vi "SingleAxisControl.vi"() -> ()   [LabVIEW 2021]
uses:
  Parameters/GetAxisParameterDouble.vi
  Parameters/GetAxisParameterString.vi
  Motion/EnableSingle.vi
  Motion/FaultAckSingle.vi
  Motion/DisableSingle.vi
  Motion/MoveIncSingle.vi
  Motion/FreerunSingle.vi
  Motion/AbortSingle.vi
  Motion/HomeSingle.vi
panel:
  in  "Disconnect?":bool
  in  "taskId":i32(ring)=1 items=["TLibrary", "T01", "T02", "T03", "T04", "T05", "T06", "T07", "T08", "T09", "T10", "T11", "T12", "T13", "T14", "T15", "T16", "T17", "T18", "T19", "T20", "T21", "T22", "T23", "T24", "T25", "T26", "T27", "T28", "T29", "T30", "T31"]
  in  "Abort":bool
  out "do stop":bool
  out "Vel Units":string
  out "Pos Units":string
  in  "stop":bool
  out "Vel Fbk":dbl
  out "Pos Fbk":dbl
  out "Status":string
  in  "Jog Right":bool
  in  "Jog Left":bool
  in  "Distance":dbl=1000.0 min=0.0 max=10.0
  in  "Speed":dbl=5000.0 min=0.0 max=100.0
  in  "Jog":bool
  in  "FaultAck":bool
  in  "Home":bool
  in  "Disable":bool
  in  "Enable":bool
  out "Axis":string
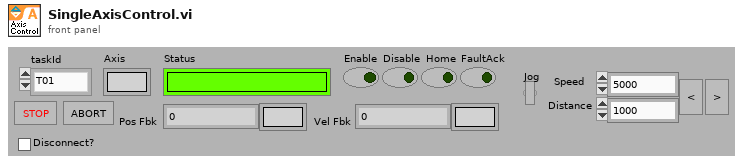
[diagram p1: front panel]
types:
  T1 = cluster{"new reference":refnum<k24>, "Event Callback":refnum<k27>, "ControllerDiagPacket":refnum<user-event>, "Event Registration Refnum":refnum<event-registration>}
  T2 = typedef "AxisDiagPacket.ctl" = cluster{"Axis Name":string, "Analog Input 0":dbl, "Analog Input 1":dbl, "Axis Fault (num)":i32, "Axis Fault (str)":string, "Axis Fault (bits)":cluster{"AmplifierFault":bool, "AmplifierTemperatureFault":bool, "CcwEndOfTravelLimitFault":bool, "CcwSoftwareLimitFault":bool, "CommunicationLostFault":bool, "CwEndOfTravelLimitFault":bool, "CwSoftwareLimitFault":bool, "EmergencyStopFault":bool, "EncoderFault":bool, "ExternalFault":bool, "FeedbackScalingFault":bool, "GantryMisalignFault ":bool, "HallSensorFault":bool, "InPositionTimeoutFault":bool, "MarkerSearchFault":bool, "MaxVelocityCommandFault":bool, "MissedInterruptFault":bool, "MotorTemperatureFault":bool, "None":bool, "OverCurrentFault":bool, "PositionErrorFault":bool, "PositionFeedbackFault":bool, "PowerSupplyFault":bool, "ProbeInputFault":bool, "SafeZoneFault":bool, "VelocityErrorFault":bool, "VelocityFeedbackFault":bool, "VoltageClampFault":bool, "InternalFault":bool}, "Axis Status (num)":i32, "Axis Status (str)":string, "Axis Status (bits)":cluster{"BacklashActive":bool, "CalibrationEnabled1D":bool, "CalibrationEnabled2D":bool, "CommandValid":bool, "DriveAbortPending":bool, "DrivePending":bool, "Enabling":bool, "GainMappingEnabled":bool, "GantryAligned":bool, "GantryRealigning":bool, "Homed":bool, "Homing":bool, "IFOVEnabled":bool, "JogGenerating":bool, "Jogging":bool, "JoystickControl":bool, "MasterSlaveControl":bool, "MotionBlocked":bool, "MotionClamped":bool, "MoveDone":bool, "None":bool, "NotVirtual":bool, "Profiling":bool, "Stability0":bool, "Stability1":bool, "TrajectoryFiltering":bool, "WaitDone":bool}, "Current Command":sgl, "Current Error":sgl, "Current Feedback":sgl, "Digital Inputs":i32, "Digital Outputs":i32, "Drive Status":i32, "Drive Status (str)":string, "Drive Status (bits)":cluster{"AccelerationPhase":bool, "AutofocusActive":bool, "BrakeOutput":bool, "CcwEndOfTravelLimitInput":bool, "CosineEncoderError":bool, "CurrentClamp":bool, "CwEndOfTravelLimitInput":bool, "DecelerationPhase":bool, "DualLoopActive":bool, "EmergencyStopInput":bool, "Enabled":bool, "EncoderClipping":bool, "GalvoCalibrationEnabled":bool, "GalvoPowerCorrection":bool, "HallAInput":bool, "HallBInput":bool, "HallCInput":bool, "HighResolutionMode":bool, "HomeLimitInput":bool, "InPosition":bool, "InPosition2":bool, "MarkerInput":bool, "MarkerLatch":bool, "MoveActive":bool, "NoMotorSupply":bool, "None":bool, "PowerLimiting":bool, "ProgrammingFlash":bool, "ProgrammingMXH":bool, "PSOHaltLatch":bool, "ServoControl":bool, "SineEncoderError":bool}, "Position Feedback Auxiliary":dbl, "Position Command":dbl, "Position Error":dbl, "Position Feedback":dbl, "Program Position Command":dbl, "Program Position Error":dbl, "Program Position Feedback":dbl, "Velocity Command":dbl, "Velocity Error":dbl, "Velocity Feedback":dbl}
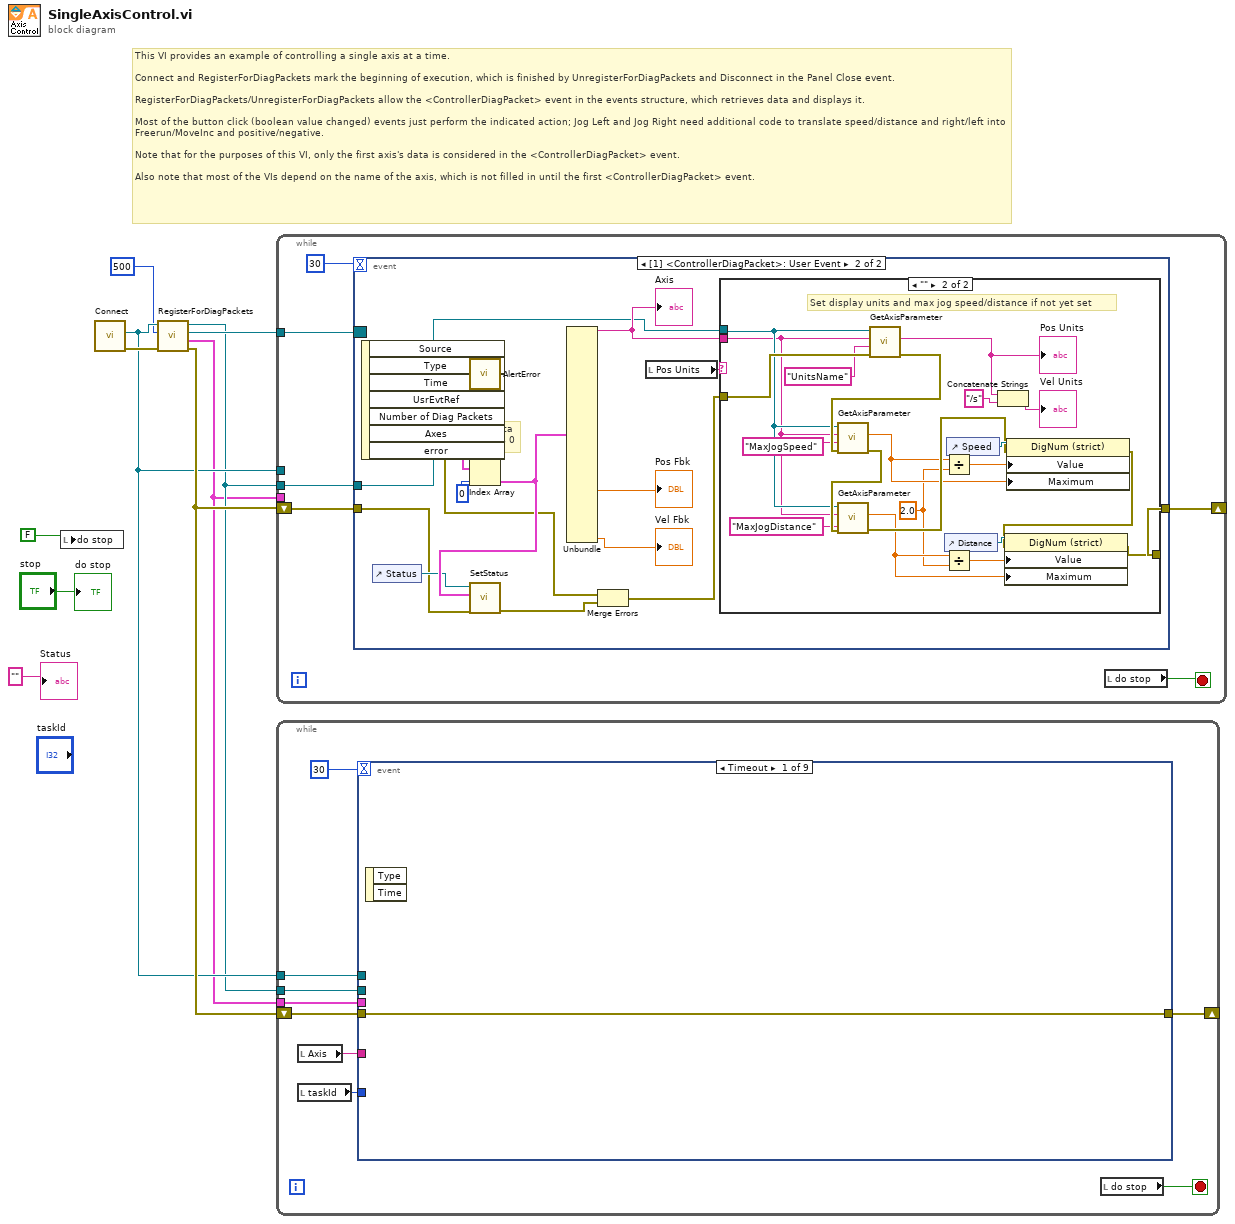
[diagram p0: block diagram]
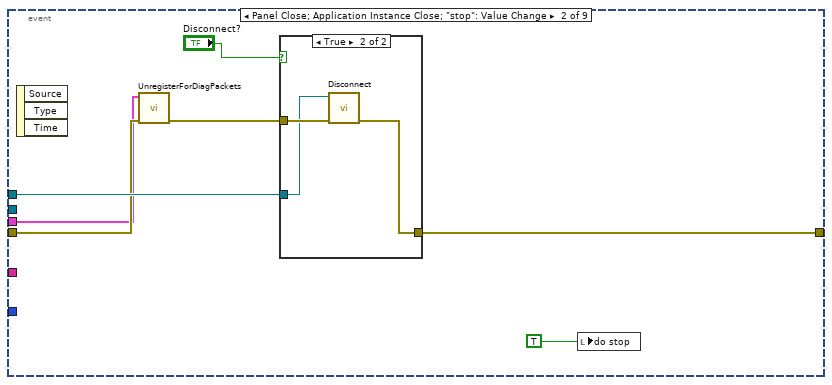
[diagram p2: hidden frame]
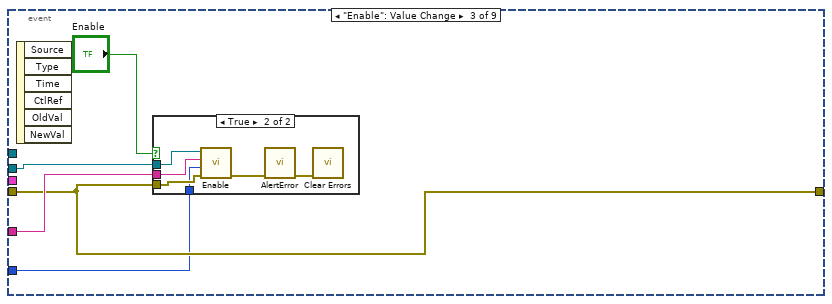
[diagram p4: hidden frame]
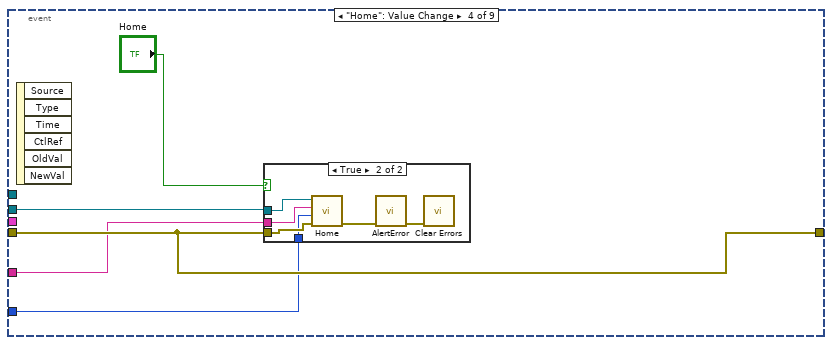
[diagram p6: hidden frame]
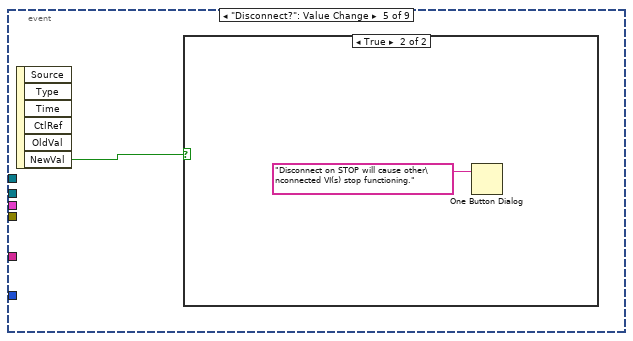
[diagram p8: hidden frame]
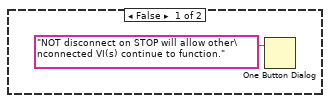
[diagram p9: hidden frame]
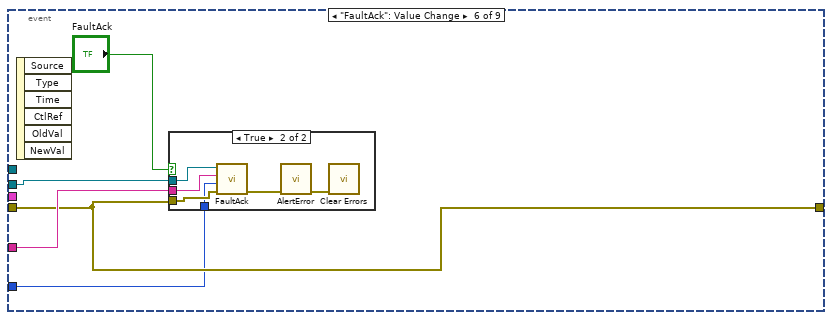
[diagram p10: hidden frame]
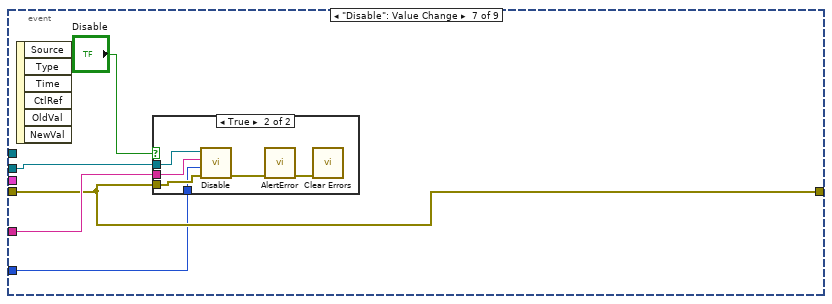
[diagram p12: hidden frame]
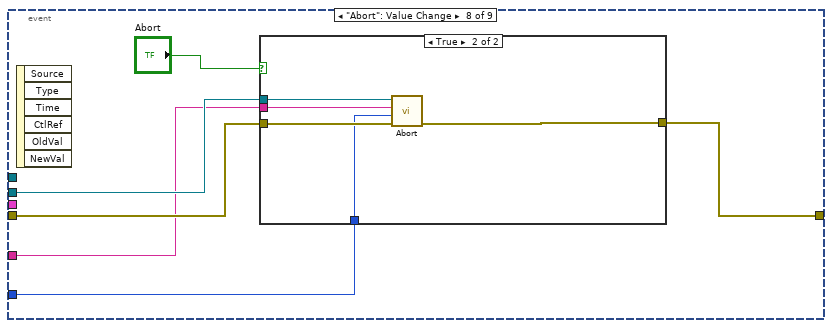
[diagram p14: hidden frame]
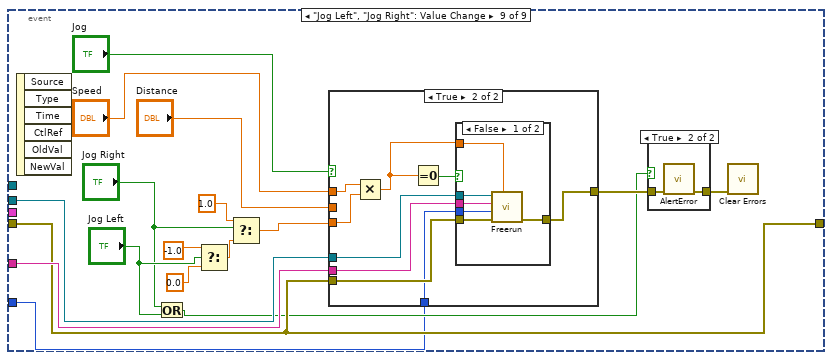
[diagram p16: hidden frame]
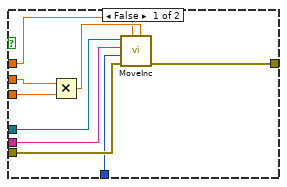
[diagram p18: hidden frame]
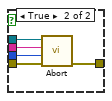
[diagram p19: hidden frame]
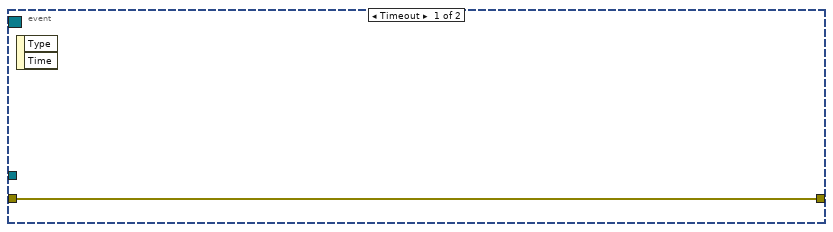
[diagram p20: hidden frame]
diagram:
  # "This VI provides an example of controlling a single axis at a time. \n\nConnect and RegisterForDiagPackets mark the beginning of execution, which is finished by UnregisterForDiagPackets and Disconnect in the Panel Close event.\n\nRegisterForDiagPackets/UnregisterForDiagPackets allow the <ControllerDiagPacket> event in the events structure, which retrieves data and displays it.\n\nMost of the button click (boolean value changed) events just perform the indicated action; Jog Left and Jog Right need additional code to translate speed/distance and right/left into Freerun/MoveInc and positive/negative.\n\nNote that for the purposes of this VI, only the first axis's data is considered in the <ControllerDiagPacket> event.\n\nAlso note that most of the VIs depend on the name of the axis, which is not filled in until the first <ControllerDiagPacket> event."
  n1 = local write "do stop"(FALSE ("do stop")) -> ()
  n2 = call "Connect.vi"() -> ("error out"=w8:errorcluster, "controller"=w4:refnum<k24>)  [unwired: 10 in]
  n3 = call "RegisterForDiagPackets.vi"("error in (no error)"=w8, "refresh interval (default)"=500, "Controller in"=w4) -> ("error out"=w7:errorcluster, "Event Metadata"=w2:T1, "Event Registration Refnum"=w10:refnum<event-registration>, "Controller out"=w3:refnum<k24>)  [unwired: 4 in]
  n4 = while {
    tunnel: w10 -> [w11]
    tunnel: w2 -> [_]
    tunnel: w3 -> [w15]
    shift-right: [w13] -> _
    shift-left: w7 -> [w14]
    tunnel: w4 -> [_]
    stop <- w12 stop-if-true
    n5 = event shown="[1] <ControllerDiagPacket>: User Event" {
      selector: w11 -> [_ _]
      dyn-events: _ -> [_ _]
      timeout: 30 -> [_ _]
      tunnel: w15 -> [_ w22]
      tunnel: w14 -> [w17 w21]
      tunnel: [w17 w20] -> w13
      event Timeout {
        n6 = event-data() -> ()  [unwired: 1 in, 2 out]
      }
      event User Event {
        # "Get data for axis 0"
        n7 = event-data() -> ("Axes"=w24:T2[], "error"=w23:errorcluster)  [unwired: 1 in, 5 out]
        n8 = control-ref of="Status"() -> (w26:refnum<vi>)
        n9 = call "AlertError.vi"("error in (no error)"=w23) -> ()  [unwired: 10 in, 1 out]
        n10 = Index Array(array=w24, index=0) -> (element=w27:T2)
        n11 = call "SetStatus.vi"("error in (no error)"=w21, "AxisDiagPacket"=w27, "Status string"=w26) -> ("error out"=w28:errorcluster)  [unwired: 8 in]
        n12 = Unbundle(w27) -> ("Axis Name"=w29:string, "Position Feedback"=→"Pos Fbk":dbl, "Velocity Feedback"=→"Vel Fbk":dbl)  [unwired: 24 out]
        "Axis" <- w29
        n13 = Merge Errors(w23, w28) -> (w30:errorcluster)
        n14 = local read "Pos Units"() -> (w31:string)
        n15 = case shown="\"\"" w31 {
          tunnel: w29 -> [_ w45]
          tunnel: w22 -> [_ w46]
          tunnel: w30 -> [w32 w50]
          tunnel: [w32 w40] -> w20
          frame Default {
          }
          frame "" {
            w33 = 2.0 ("y")
            # "Set display units and max jog speed/distance if not yet set"
            n16 = call-poly "GetAxisParameter.vi"("error in (no error)"=w50, "Parameter Name"="UnitsName" ("parameter name"), "axis name"=w45, "controller in"=w46) -> ("error out"=w47:errorcluster, "value"=w51:string)  [unwired: 5 in, 1 out]
            "Pos Units" <- w51
            n17 = call-poly "GetAxisParameter.vi"("error in (no error)"=w47, "Parameter Name"="MaxJogSpeed" ("parameter name"), "axis name"=w45, "controller in"=w46) -> ("error out"=w48:errorcluster, "value"=w35:dbl)  [unwired: 5 in, 1 out]
            n18 = call-poly "GetAxisParameter.vi"("error in (no error)"=w48, "Parameter Name"="MaxJogDistance" ("parameter name"), "axis name"=w45, "controller in"=w46) -> ("error out"=w38:errorcluster, "value"=w34:dbl)  [unwired: 5 in, 1 out]
            n19 = Divide(x=w35, y=w33) -> (x/y=w36:dbl)
            n20 = Divide(x=w34, y=w33) -> (x/y=w37:dbl)
            n21 = control-ref of="Distance"() -> (w41:refnum<vi>)
            n22 = control-ref of="Speed"() -> (w42:refnum<vi>)
            n23 = Concatenate Strings(w51, "/s" ("string")) -> (→"Vel Units":string)
            n24 = property class="DigNum (strict)"(reference=w42, error in=w38, "Value"=w36, "Maximum"=w35) -> (error out=w39:errorcluster)  [unwired: 1 out]
            n25 = property class="DigNum (strict)"(reference=w41, error in=w39, "Value"=w37, "Maximum"=w34) -> (error out=w40:errorcluster)  [unwired: 1 out]
          }
        }
      }
    }
    n26 = local read "do stop"() -> (w12:bool)
  }
  n27 = while {
    tunnel: w4 -> [w62]
    tunnel: w3 -> [w56]
    shift-right: [w57] -> _
    shift-left: w7 -> [w61]
    tunnel: w2 -> [w55]
    stop <- w58 stop-if-true
    n28 = local read "Axis"() -> (w60:string)
    n29 = local read "taskId"() -> (w54:i32)
    n30 = event shown="[0] Timeout" {
      selector: _ -> [_ _ _ _ _ _ _ _ _]
      dyn-events: _ -> [_ _ _ _ _ _ _ _ _]
      timeout: 30 -> [_ _ _ _ _ _ _ _ _]
      tunnel: w56 -> [_ _ w79 w86 _ w104 w114 w125 w141]
      tunnel: w61 -> [w63 w65 w76 w90 _ w102 w112 w126 w140]
      tunnel: [w63 w70 w76 w90 _ w102 w112 w124 w140] -> w57
      tunnel: w60 -> [_ _ w78 w89 _ w103 w113 w123 w142]
      tunnel: w62 -> [_ w69 _ _ _ _ _ _ _]
      tunnel: w55 -> [_ w64 _ _ _ _ _ _ _]
      tunnel: w54 -> [_ _ w75 w88 _ w100 w111 w122 w134]
      event Timeout {
        n31 = event-data() -> ()  [unwired: 1 in, 2 out]
      }
      event Panel Close; Application Instance Close; "stop": Value Change {
        n32 = event-data() -> ()  [unwired: 1 in, 3 out]
        n33 = call "UnregisterForDiagPackets.vi"("Event Metadata"=w64, "error in (no error)"=w65) -> ("error out"=w66:errorcluster)  [unwired: 8 in]
        n34 = case shown="True" "Disconnect?" {
          tunnel: w66 -> [w71 w74]
          tunnel: [w71 w73] -> w70
          tunnel: w69 -> [_ w72]
          frame False {
          }
          frame True {
            n35 = call "Disconnect.vi"("error in (no error)"=w74, "controller"=w72) -> ("error out"=w73:errorcluster)  [unwired: 9 in]
          }
        }
        n36 = local write "do stop"(TRUE) -> ()
      }
      event "Enable": Value Change {
        n37 = event-data() -> ()  [unwired: 1 in, 6 out]
        n38 = case shown="True" "Enable" {
          tunnel: w79 -> [_ w84]
          tunnel: w76 -> [_ w82]
          tunnel: w78 -> [_ w83]
          tunnel: w75 -> [_ w80]
          frame False {
          }
          frame True {
            n39 = call-poly "Enable.vi"("error in (no error)"=w82, "taskId"=w80, "axis name"=w83, "controller in"=w84) -> ("error out"=w81:errorcluster)  [unwired: 6 in, 1 out]
            n40 = call "AlertError.vi"("error in (no error)"=w81) -> ("error out"=w85:errorcluster)  [unwired: 10 in]
            n41 = call <vilib>:"Clear Errors.vi"("error in (no error)"=w85) -> ()  [unwired: 5 in, 2 out]
          }
        }
      }
      event "Home": Value Change {
        n42 = event-data() -> ()  [unwired: 1 in, 6 out]
        n43 = case shown="True" "Home" {
          tunnel: w86 -> [_ w96]
          tunnel: w90 -> [_ w94]
          tunnel: w89 -> [_ w95]
          tunnel: w88 -> [_ w91]
          frame False {
          }
          frame True {
            n44 = call-poly "Home.vi"("error in (no error)"=w94, "taskId"=w91, "axis name"=w95, "controller in"=w96) -> ("error out"=w93:errorcluster)  [unwired: 6 in, 1 out]
            n45 = call "AlertError.vi"("error in (no error)"=w93) -> ("error out"=w92:errorcluster)  [unwired: 10 in]
            n46 = call <vilib>:"Clear Errors.vi"("error in (no error)"=w92) -> ()  [unwired: 5 in, 2 out]
          }
        }
      }
      event "Disconnect?": Value Change {
        n47 = event-data() -> ("NewVal"=w97:bool)  [unwired: 1 in, 5 out]
        n48 = case shown="True" w97 {
          frame False {
            n49 = One Button Dialog(message="NOT disconnect on STOP will allow other\nconnected VI(s) continue to function.") -> ()  [unwired: 1 in, 1 out]
          }
          frame True {
            n50 = One Button Dialog(message="Disconnect on STOP will cause other\nconnected VI(s) stop functioning.") -> ()  [unwired: 1 in, 1 out]
          }
        }
      }
      event "FaultAck": Value Change {
        n51 = event-data() -> ()  [unwired: 1 in, 6 out]
        n52 = case shown="True" "FaultAck" {
          tunnel: w104 -> [_ w110]
          tunnel: w102 -> [_ w108]
          tunnel: w103 -> [_ w109]
          tunnel: w100 -> [_ w105]
          frame False {
          }
          frame True {
            n53 = call-poly "FaultAck.vi"("error in (no error)"=w108, "taskId"=w105, "axis name"=w109, "controller in"=w110) -> ("error out"=w107:errorcluster)  [unwired: 6 in, 1 out]
            n54 = call "AlertError.vi"("error in (no error)"=w107) -> ("error out"=w106:errorcluster)  [unwired: 10 in]
            n55 = call <vilib>:"Clear Errors.vi"("error in (no error)"=w106) -> ()  [unwired: 5 in, 2 out]
          }
        }
      }
      event "Disable": Value Change {
        n56 = event-data() -> ()  [unwired: 1 in, 6 out]
        n57 = case shown="True" "Disable" {
          tunnel: w114 -> [_ w121]
          tunnel: w112 -> [_ w119]
          tunnel: w113 -> [_ w120]
          tunnel: w111 -> [_ w116]
          frame False {
          }
          frame True {
            n58 = call-poly "Disable.vi"("error in (no error)"=w119, "taskId"=w116, "axis name"=w120, "controller in"=w121) -> ("error out"=w118:errorcluster)  [unwired: 6 in, 1 out]
            n59 = call "AlertError.vi"("error in (no error)"=w118) -> ("error out"=w117:errorcluster)  [unwired: 10 in]
            n60 = call <vilib>:"Clear Errors.vi"("error in (no error)"=w117) -> ()  [unwired: 5 in, 2 out]
          }
        }
      }
      event "Abort": Value Change {
        n61 = event-data() -> ()  [unwired: 1 in, 6 out]
        n62 = case shown="True" "Abort" {
          tunnel: w125 -> [_ w133]
          tunnel: w126 -> [w128 w132]
          tunnel: [w128 w131] -> w124
          tunnel: w123 -> [_ w130]
          tunnel: w122 -> [_ w129]
          frame False {
          }
          frame True {
            n63 = call-poly "Abort.vi"("error in (no error)"=w132, "taskId"=w129, "axis name? (all)"=w130, "controller in"=w133) -> ("error out"=w131:errorcluster)  [unwired: 6 in, 1 out]
          }
        }
      }
      event "Jog Left", "Jog Right": Value Change {
        n64 = event-data() -> ()  [unwired: 1 in, 6 out]
        n65 = Or(x="Jog Right", y="Jog Left") -> (x .or. y?=w135:bool)
        n66 = Select(t=-1.0, s="Jog Left", f=0.0) -> (s? t:f=w150:dbl)
        n67 = Select(t=1.0, s="Jog Right", f=w150) -> (s? t:f=w146:dbl)
        n68 = case shown="True" "Jog" {
          tunnel: "Speed" -> [w157 w171]
          tunnel: "Distance" -> [w162 _]
          tunnel: w146 -> [w161 w170]
          tunnel: w140 -> [w160 w169]
          tunnel: w142 -> [w156 w168]
          tunnel: w141 -> [w155 w167]
          tunnel: [w159 w166] -> w138
          tunnel: w134 -> [w154 w165]
          frame False {
            n69 = Multiply(x=w162, y=w161) -> (x*y=w158:dbl)
            n70 = call-poly "MoveInc.vi"("distance"=w158, "speed"=w157, "error in (no error)"=w160, "taskId"=w154, "axis name"=w156, "controller in"=w155) -> ("error out"=w159:errorcluster)  [unwired: 4 in, 1 out]
          }
          frame True {
            n71 = Multiply(x=w171, y=w170) -> (x*y=w163:dbl)
            n72 = Equal To 0?(x=w163) -> (x = 0?=w164:bool)
            n73 = case shown="False" w164 {
              tunnel: w169 -> [w177 w182]
              tunnel: w168 -> [w176 w179]
              tunnel: w167 -> [w175 w180]
              tunnel: [w174 w181] -> w166
              tunnel: w163 -> [w173 _]
              tunnel: w165 -> [w172 w178]
              frame False {
                n74 = call-poly "Freerun.vi"("speed"=w173, "error in (no error)"=w177, "taskId"=w172, "axis name"=w176, "controller in"=w175) -> ("error out"=w174:errorcluster)  [unwired: 5 in, 1 out]
              }
              frame True {
                n75 = call-poly "Abort.vi"("error in (no error)"=w182, "taskId"=w178, "axis name? (all)"=w179, "controller in"=w180) -> ("error out"=w181:errorcluster)  [unwired: 6 in, 1 out]
              }
            }
          }
        }
        n76 = case shown="True" w135 {
          tunnel: [w151 w153] -> w139
          tunnel: w138 -> [w151 w152]
          frame False {
          }
          frame True {
            n77 = call "AlertError.vi"("error in (no error)"=w152) -> ("error out"=w153:errorcluster)  [unwired: 10 in]
          }
        }
        n78 = call <vilib>:"Clear Errors.vi"("error in (no error)"=w139) -> ()  [unwired: 5 in, 2 out]
      }
    }
    n79 = local read "do stop"() -> (w58:bool)
  }
  "Status" <- "" ("Status")
  "do stop" <- "stop"
